vi "Periodic Tasks.vi"(8 "error in":errorcluster) -> ()   [LabVIEW 2020]
doc: "This VI runs in parallel to other tasks. It can contain as many user-defined periodic loops as you need. These can carry out PID or other sorts of timed response."
uses:
  <vilib>/Rock Robotics/WPI/ThirdParty/Phoenix-LabVIEW/Motor Controller/Controls/CTRE_Phoenix_MotorControl_ControlMode.ctl
  <vilib>/Rock Robotics/WPI/ThirdParty/Sensors/navX/_TypeDefs/FRIC_navX_DeviceNumbersTypeDef.ctl
  <vilib>/Rock Robotics/SystemInterfaces/i2clib/i2c_bus.ctl
  <vilib>/Rock Robotics/Network Tables/NT Read Boolean.vi
  <vilib>/Rock Robotics/WPI/ThirdParty/Sensors/navX/_Processing Loop/FRIC_navX_Internal_I2C_ProcessingLoop.vi
  Robot Global Data.vi
  <vilib>/Rock Robotics/Network Tables/NT Read String.vi
panel:
  in  "Tab Control":enum32{"Page 1"}(tab)
  in  "list of Falcon 500 RefNum":string[](array[string])=["DriveLEFT", "DriveRIGHT", "SHOOTER", "INTAKE DRIVE", "ClimberLEFT", "ClimberRIGHT"]
  in  "list of NEO RefNum":string[](array[string])=["INTAKE LIFT", "ARMLEFT", "ARMRIGHT"]
  out "LEFT MATCHED?":bool
  out "RIGHT MATCHED?":bool
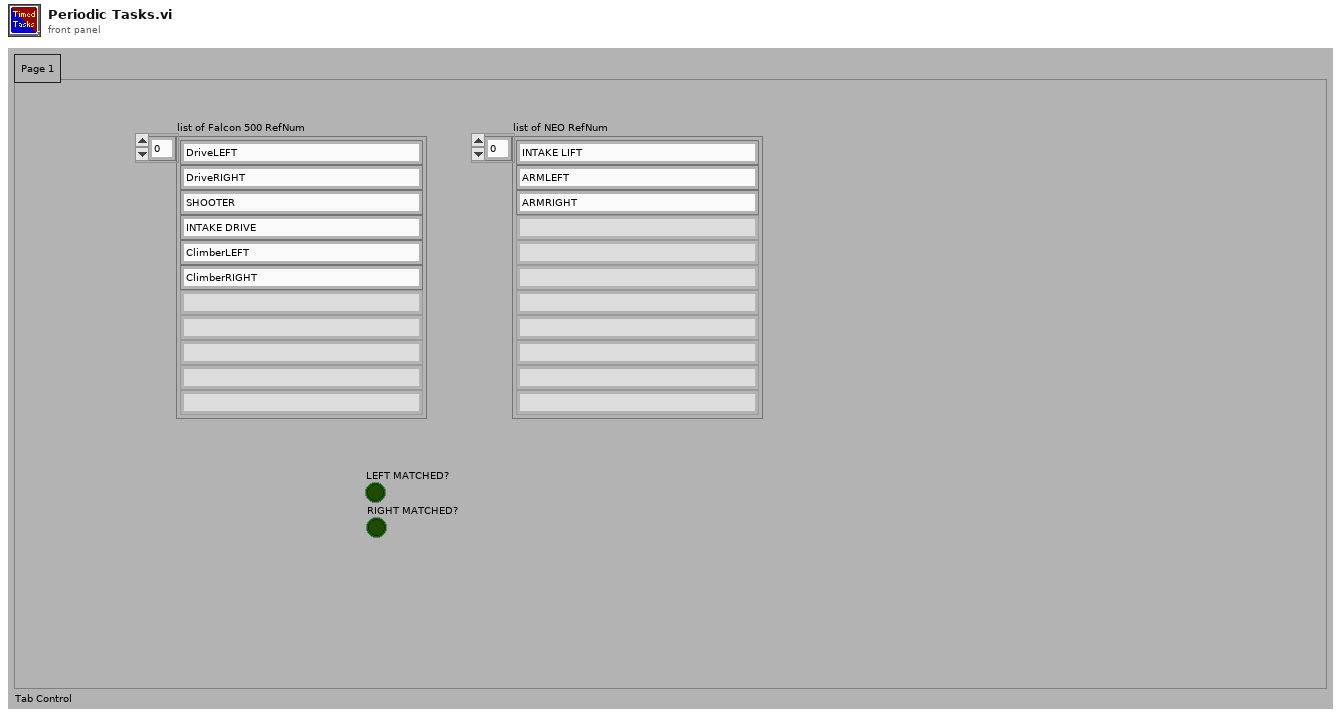
[diagram p1: front panel]
types:
  T1 = typedef "i2c_bus.ctl" = enum16{"I2C On-Board", "I2C MXP", "Invalid"}
  T2 = typedef "FRIC_navX_DeviceNumbersTypeDef.ctl" = enum16{"Dev0", "Dev1", "Dev2", "Dev3"}
  T3 = typedef "WPI_AccelerometerDevRef.ctl" = cluster{"DevStatus":errorcluster, "Scaling":T4, "Analog Channels":T5, "I2C Bus":T1, "SPI Bus":T7, "Accel Range":T8, "ADXL Axes":T9, "Handle":i32, "Device Address":u8, "Accel Type":enum16{"Analog", "ADXL345 I2C", "ADXL345 SPI", "Internal", "ADXL362 SPI"}}
  T4 = typedef "WPI_AccelerometerScaling.ctl" = cluster{"Gain (VoltsPerG)":dbl, "Center Voltage":dbl}
  T5 = typedef "WPI_AccelerometerAnalogChannels.ctl" = cluster{"X-Axis":T6, "Y-Axis":T6, "Z-Axis":T6}
  T6 = typedef "FPGA_AIChannel.ctl" = enum8{"AI 0", "AI 1", "AI 2", "AI 3", "AI MXP 0", "AI MXP 1", "AI MXP 2", "AI MXP 3", "Invalid"}
  T7 = typedef "spi_bus.ctl" = enum16{"SPI On-Board, CS0", "SPI On-Board, CS1", "SPI On-Board, CS2", "SPI On-Board, CS3", "SPI MXP", "Invalid"}
  T8 = typedef "ADXL345 Range.ctl" = u8
  T9 = typedef "WPI_AccelerometerADXL345 Axes.ctl" = cluster{"X-Axis":bool, "Y-Axis":bool, "Z-Axis":bool}
  T10 = typedef "WPI_MotorControlDeviceRef.ctl" = cluster{"DeviceStatus":errorcluster, "Type":T11, "PWM":cluster{"PWM Channel":T12, "DeadBand":T13}, "CAN":cluster{"Device Number":u8, "SetOutput VI Ref":variant, "GetOutput VI Ref":variant, "Enable VI Ref":variant, "Disable VI Ref":variant, "Data":variant}, "Invert":bool, "DIO PWM":cluster{"PWM \"Enable\" Channel":T12, "DIOChannel":T14, "PWM Rate":dbl}}
  T11 = typedef "WPI_MotorControlType.ctl" = enum16{"PWM", "CAN", "DIO PWM"}
  T12 = typedef "FPGA_DIOPWMChannel.ctl" = enum8{"PWM 0", "PWM 1", "PWM 2", "PWM 3", "PWM 4", "PWM 5", "PWM 6", "PWM 7", "PWM 8", "PWM 9", "PWM MXP 0", "PWM MXP 1", "PWM MXP 2", "PWM MXP 3", "PWM MXP 4", "PWM MXP 5", "PWM MXP 6", "PWM MXP 7", "PWM MXP 8", "PWM MXP 9", "Invalid"}
  T13 = typedef "WPI_PWMDeadband.ctl" = cluster{"Name":string, "maxPositivePwm":i32, "minPositivePwm":i32, "centerPwm":i32, "maxNegativePwm":i32, "minNegativePwm":i32, "angularRange":u16}
  T14 = typedef "FPGA_DIOChannel.ctl" = enum8{"DIO 0", "DIO 1", "DIO 2", "DIO 3", "DIO 4", "DIO 5", "DIO 6", "DIO 7", "DIO 8", "DIO 9", "DIO MXP 0", "DIO MXP 1", "DIO MXP 2", "DIO MXP 3", "DIO MXP 4", "DIO MXP 5", "DIO MXP 6", "DIO MXP 7", "DIO MXP 8", "DIO MXP 9", "DIO MXP 10", "DIO MXP 11", "DIO MXP 12", "DIO MXP 13", "DIO MXP 14", "DIO MXP 15", "SPI Port CS1", "SPI Port CS2", "SPI Port CS3", "SPI Port MISO", "SPI Port MOSI", "Invalid"}
  T15 = cluster{"planetary gear ratio:1":i32, "GEAR TEETH on planetary":i32, "GEAR TEETH on lift arm":i32, "convert motor revs to lift degrees":dbl, "MIN (deg)":dbl, "MAX (deg)":dbl, "roller speed%":dbl, "tip over (deg)":dbl, "lift speed% EXTEND":dbl, "lift speed% RETRACT":dbl}
  T16 = typedef "CTRE_Phoenix_MotorControl_ControlMode.ctl" = u16
  T17 = cluster{"POSITION?":bool, "LIMITS?":bool, "TEMP?":bool, "ELECT?":bool, "INTSENSOR?":bool}
  T18 = cluster{"POSITION?":bool, "LIMITS?":bool, "TEMP?":bool, "ELECT?":bool}
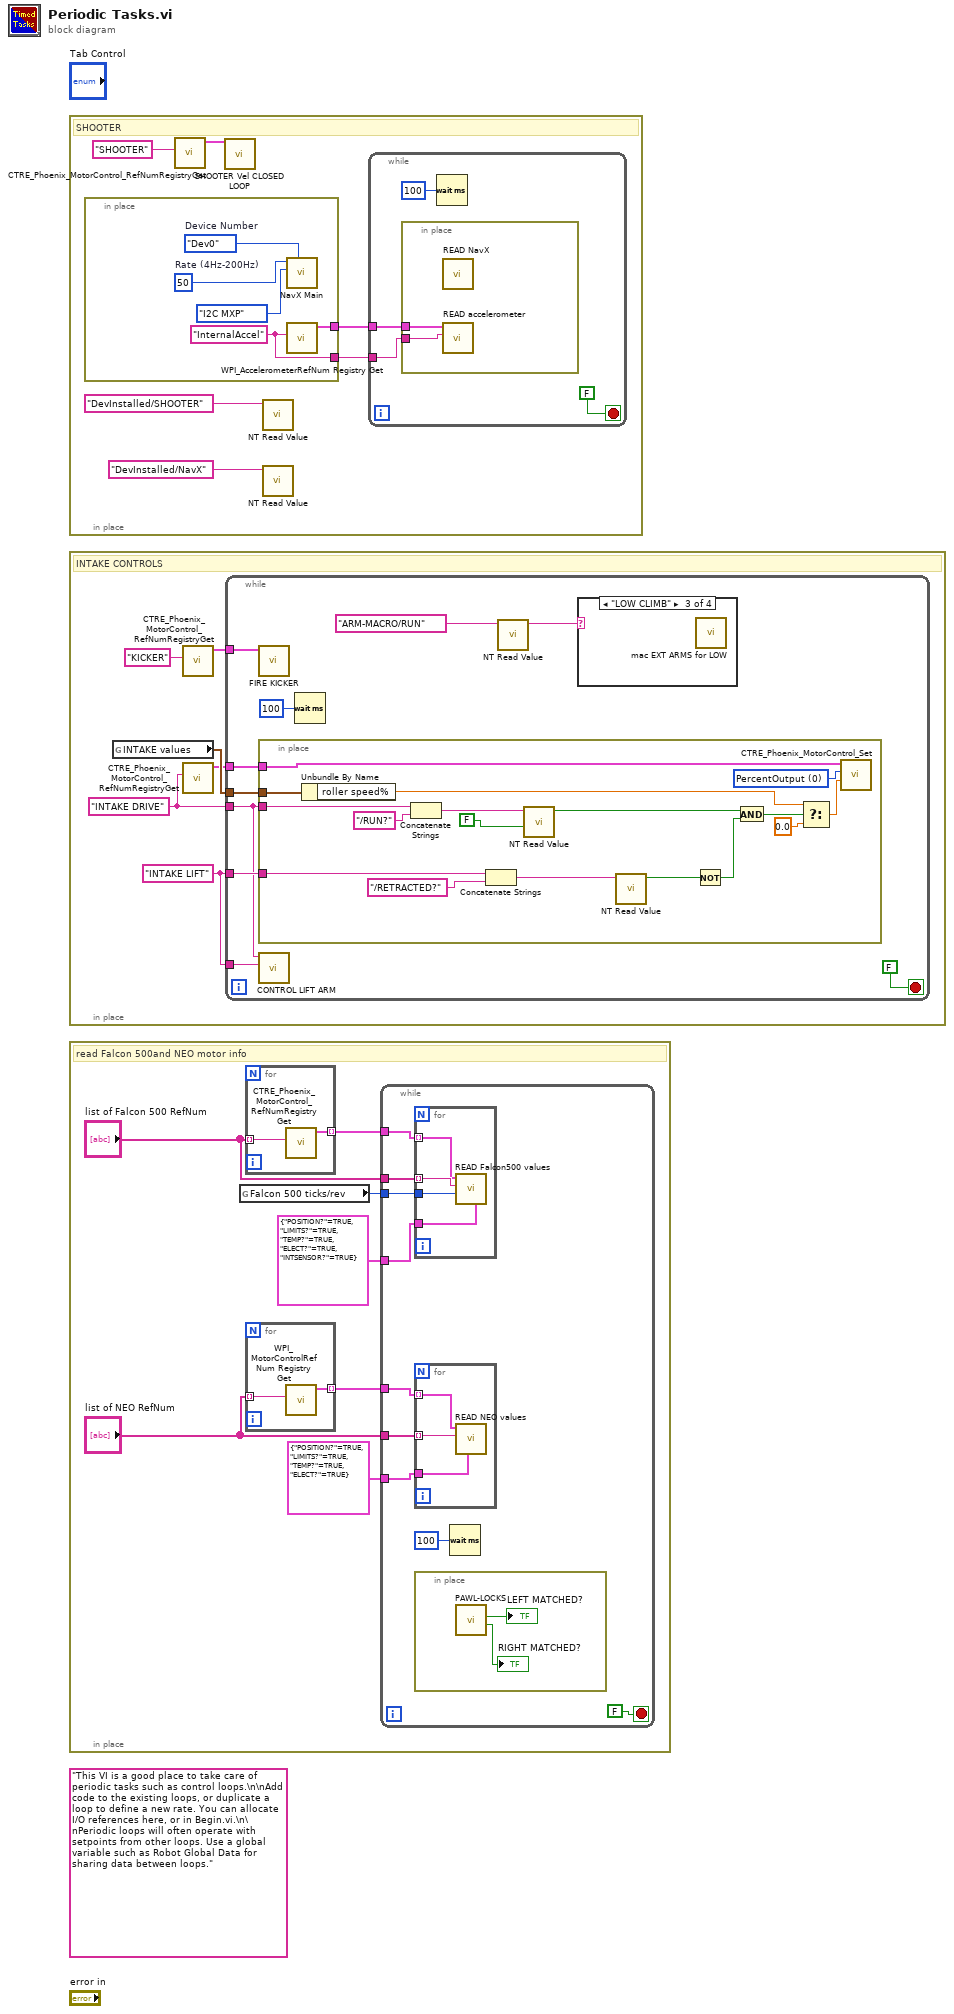
[diagram p0: block diagram]
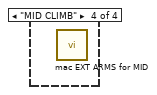
[diagram p4: hidden frame]
diagram:
  (unwired) "This VI is a good place to take care of periodic tasks such as control loops.\n\nAdd code to the existing loops, or duplicate a loop to define a new rate. You can allocate I/O references here, or in Begin.vi.\n\nPeriodic loops will often operate with setpoints from other loops. Use a global variable such as Robot Global Data for sharing data between loops."
  n1 = in-place {
    # "SHOOTER"
    n2 = in-place {
      in-place-border: [w8] -> w4
      in-place-border: [w7] -> w3
      w7 = "InternalAccel" ("refnum name")
      w10 = u8 50  # Rate (4Hz-200Hz)
      w11 = FRIC_navX_DeviceNumbersTypeDef."Dev0"  # Device Number
      n3 = call-poly <vilib>:"NavX Main.vi"("Device Number"=w11, "I2C Bus"=i2c_bus."I2C MXP", "Rate (4Hz-200Hz)"=w10) -> ()  [unwired: 9 in]
      n4 = call <vilib>:"WPI_AccelerometerRefNum Registry Get.vi"("refnum name"=w7) -> ("AccelerometerDevRef"=w8:T3)  [unwired: 9 in, 1 out]
    }
    n5 = call <vilib>:"CTRE_Phoenix_MotorControl_RefNumRegistryGet.vi"("refnum name"="SHOOTER") -> ("PhoenixMotorControlDevRef"=w1:T10)  [unwired: 9 in, 1 out]
    n6 = call "SHOOTER Vel CLOSED LOOP.vi"("PhoenixMotorControlDevRef IN"=w1) -> ()  [unwired: 16 in, 3 out]
    n7 = call-poly <vilib>:"NT Read Value.vi"("Name"="DevInstalled/SHOOTER") -> ()  [unwired: 9 in, 2 out]
    n8 = call-poly <vilib>:"NT Read Value.vi"("Name"="DevInstalled/NavX") -> ()  [unwired: 9 in, 2 out]
    n9 = while {
      tunnel: w4 -> [w13]
      tunnel: w3 -> [w12]
      stop <- FALSE stop-if-true
      n10 = in-place {
        in-place-border: w13 -> [w17]
        in-place-border: w12 -> [w16]
        n11 = call "READ NavX.vi"() -> ()  [unwired: 10 in, 2 out]
        n12 = call "READ accelerometer.vi"("refnum name"=w16, "AccelerometerDevRef"=w17) -> ()  [unwired: 10 in]
      }
      n13 = Wait (ms)(milliseconds to wait=u32 100) -> ()  [unwired: 1 out]
    }
  }
  n14 = in-place {
    w20 = "INTAKE LIFT" ("string")
    w21 = "INTAKE DRIVE" ("string")
    # "INTAKE CONTROLS"
    n15 = global read "Robot Global Data.vi" "INTAKE values"() -> (w23:T15)
    n16 = call <vilib>:"CTRE_Phoenix_MotorControl_RefNumRegistryGet.vi"("refnum name"="KICKER") -> ("PhoenixMotorControlDevRef"=w18:T10)  [unwired: 9 in, 1 out]
    n17 = call <vilib>:"CTRE_Phoenix_MotorControl_RefNumRegistryGet.vi"("refnum name"=w21) -> ("PhoenixMotorControlDevRef"=w22:T10)  [unwired: 9 in, 1 out]
    n18 = while {
      tunnel: w21 -> [w27]
      tunnel: w23 -> [w31]
      tunnel: w20 -> [w29]
      tunnel: w20 -> [w28]
      tunnel: w22 -> [w30]
      tunnel: w18 -> [w26]
      stop <- FALSE stop-if-true
      n19 = call "FIRE KICKER.vi"("VictorSPX devref in"=w26) -> ()  [unwired: 9 in, 2 out]
      n20 = in-place {
        in-place-border: w27 -> [w47]
        in-place-border: w31 -> [w46]
        in-place-border: w30 -> [w43]
        in-place-border: w28 -> [w41]
        w44 = T16 0 items=["PercentOutput"=0, "Position"=1, "Velocity"=2, "Current"=3, "Follower"=5, "MotionProfile"=6, "MotionMagic"=7, "MotionProfileArc"=10, "Disabled"=15] ("Control Mode")
        n21 = Unbundle By Name(w46) -> ("roller speed%"=w45:dbl)
        n22 = Concatenate Strings(w47, "/RUN?" ("Name")) -> (w49:string)
        n23 = Concatenate Strings(w41, "/RETRACTED?" ("string")) -> (w40:string)
        n24 = call-poly <vilib>:"NT Read Value.vi"("Default Value"=FALSE, "Name"=w49) -> ("Boolean"=w36:bool)  [unwired: 8 in, 1 out]
        n25 = call-poly <vilib>:"NT Read Value.vi"("Name"=w40) -> ("Boolean"=w35:bool)  [unwired: 9 in, 1 out]
        n26 = Not(x=w35) -> (.not. x?=w34:bool)
        n27 = And(x=w36, y=w34) -> (x .and. y?=w37:bool)
        n28 = Select(t=w45, s=w37, f=0.0) -> (s? t:f=w42:dbl)
        n29 = call <vilib>:"CTRE_Phoenix_MotorControl_Set.vi"("Output"=w42, "Control Mode"=w44, "PhoenixMotorControlDevRef"=w43) -> ()  [unwired: 7 in, 2 out]
      }
      n30 = call "CONTROL LIFT ARM.vi"("LIFT ARM refname"=w29, "LIFT DRIVE refname"=w27) -> ()  [unwired: 9 in, 1 out]
      n31 = Wait (ms)(milliseconds to wait=u32 100) -> ()  [unwired: 1 out]
      n32 = call-poly <vilib>:"NT Read Value.vi"("Name"="ARM-MACRO/RUN") -> ("String"=w24:string)  [unwired: 9 in, 1 out]
      n33 = case shown="\"LOW CLIMB\"" w24 {
        frame "False" {
        }
        frame "", Default {
        }
        frame "LOW CLIMB" {
          n34 = call "mac EXT ARMS for LOW.vi"() -> ()  [unwired: 11 in, 1 out]
        }
        frame "MID CLIMB" {
          n35 = call "mac EXT ARMS for MID.vi"() -> ()  [unwired: 11 in, 1 out]
        }
      }
    }
  }
  n36 = in-place {
    # "read Falcon 500and NEO motor info"
    n37 = global read "Robot Global Data.vi" "Falcon 500 ticks/rev"() -> (w55:i32)
    n38 = for {
      tunnel: "list of Falcon 500 RefNum" -> [w61] mode=indexing
      tunnel: [w60] -> w57 mode=indexing
      n39 = call <vilib>:"CTRE_Phoenix_MotorControl_RefNumRegistryGet.vi"("refnum name"=w61) -> ("PhoenixMotorControlDevRef"=w60:T10)  [unwired: 9 in, 1 out]
    }
    n40 = for {
      tunnel: "list of NEO RefNum" -> [w59] mode=indexing
      tunnel: [w58] -> w54 mode=indexing
      n41 = call <vilib>:"WPI_MotorControlRefNum Registry Get.vi"("refnum name"=w59) -> ("MotorControlDevRef"=w58:T10)  [unwired: 9 in, 1 out]
    }
    n42 = while {
      tunnel: w57 -> [w68]
      tunnel: "list of Falcon 500 RefNum" -> [w67]
      tunnel: w55 -> [w66]
      tunnel: w54 -> [w65]
      tunnel: "list of NEO RefNum" -> [w64]
      tunnel: T18 {"POSITION?"=TRUE, "LIMITS?"=TRUE, "TEMP?"=TRUE, "ELECT?"=TRUE} ("NEO data switches") -> [w63]
      tunnel: T17 {"POSITION?"=TRUE, "LIMITS?"=TRUE, "TEMP?"=TRUE, "ELECT?"=TRUE, "INTSENSOR?"=TRUE} ("FALCON data switches") -> [w62]
      stop <- FALSE stop-if-true
      n43 = for {
        tunnel: w68 -> [w78] mode=indexing
        tunnel: w67 -> [w79] mode=indexing
        tunnel: w66 -> [w77]
        tunnel: w62 -> [w76]
        n44 = call "READ Falcon500 values.vi"("PhoenixMotorControlDevRef"=w78, "refnum name"=w79, "ticks per rev"=w77, "FALCON data switches"=w76) -> ()  [unwired: 4 in, 2 out]
      }
      n45 = for {
        tunnel: w65 -> [w74] mode=indexing
        tunnel: w64 -> [w75] mode=indexing
        tunnel: w63 -> [w73]
        n46 = call "READ NEO values.vi"("NEO data switches"=w73, "RefName"=w75, "MotorControlDevRef"=w74) -> ()  [unwired: 7 in, 2 out]
      }
      n47 = in-place {
        n48 = call "PAWL-LOCKS.vi"() -> ("RIGHT MATCHED?"=→"RIGHT MATCHED?":bool, "LEFT MATCHED?"=→"LEFT MATCHED?":bool)  [unwired: 9 in, 1 out]
      }
      n49 = Wait (ms)(milliseconds to wait=u32 100) -> ()  [unwired: 1 out]
    }
  }
